vi "Waterfall Constructor.vi"(4 "Plot ID":i32, 6 "z matrix":sgl[][](array[numeric]), 8 "error in (no error)":errorcluster, 9 "y matrix":sgl[][](array[numeric]), 10 "x matrix":sgl[][](array[numeric]), 11 "3D Waterfall Datatype.lvclass in":refnum<class "3D Waterfall Datatype.lvclass">) -> (0 "error out":errorcluster, 3 "3D Waterfall Datatype.lvclass out":refnum<class "3D Waterfall Datatype.lvclass">)   [LabVIEW 2020, in "3D Waterfall Datatype.lvclass"]
uses:
  <vilib>/Math Plots/3D Math Plots/3D Waterfall/3D Waterfall Datatype/3D Waterfall Datatype.lvclass
  <vilib>/Math Plots/3D Math Plots/3D Waterfall/3D Waterfall Datatype/3D Waterfall Datatype.lvclass/3D Waterfall Datatype.ctl
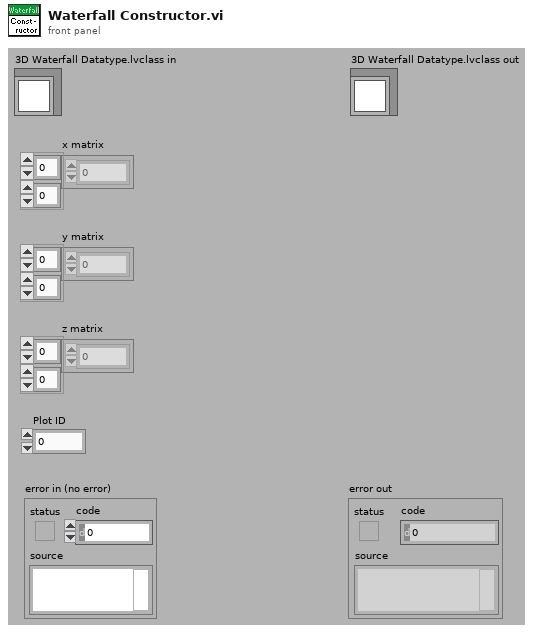
[diagram p1: front panel]
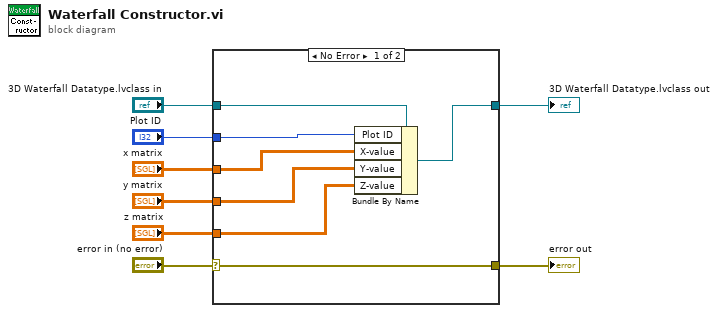
[diagram p0: block diagram]
diagram:
  n1 = case shown="No Error" "error in (no error)" {
    selector: "error in (no error)" -> [w10 w17]
    tunnel: "Plot ID" -> [w9 _]
    tunnel: [w10 w17] -> w7
    tunnel: "x matrix" -> [w15 _]
    tunnel: "y matrix" -> [w14 _]
    tunnel: "z matrix" -> [w13 _]
    tunnel: "3D Waterfall Datatype.lvclass in" -> [w12 w16]
    tunnel: [w11 w16] -> w1
    frame No Error {
      n2 = Bundle By Name(cluster=w12, "Plot ID"=w9, "X-value"=w15, "Y-value"=w14, "Z-value"=w13) -> (w11:refnum<class "3D Waterfall Datatype.lvclass">)
    }
    frame Error {
    }
  }
  "error out" <- w7
  "3D Waterfall Datatype.lvclass out" <- w1
